vi "Remove Tildes (Array).vi"(3 "String In":string[](array[string])) -> (1 "String Out":string[](array[string]))   [LabVIEW 2019]
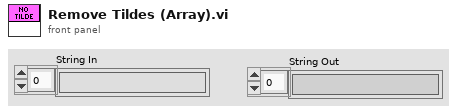
[diagram p1: front panel]
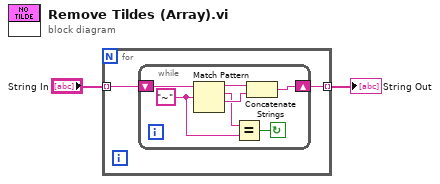
[diagram p0: block diagram]
diagram:
  n1 = for {
    tunnel: "String In" -> [w4] mode=indexing
    tunnel: [w3] -> w1 mode=indexing
    n2 = while {
      shift-right: [w8] -> w3
      shift-left: w4 -> [w11]
      stop <- w5 continue-if-true
      w7 = "~" ("regular expression")
      n3 = Match Pattern(string=w11, regular expression=w7) -> (before substring=w10:string, match substring=w6:string, after substring=w9:string)  [unwired: 1 in, 1 out]
      n4 = Equal?(x=w6, y=w7) -> (x = y?=w5:bool)
      n5 = Concatenate Strings(w10, w9) -> (w8:string)
    }
  }
  "String Out" <- w1
